vi "Potting Main.vi"   [LabVIEW 2011]
uses:
  Shared Components/Gantry Class/Gantry Class.lvclass
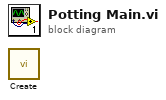
[diagram p0: block diagram]
diagram:
  n1 = call "Create.vi"() -> ()  [unwired: 10 in, 2 out]
